vi "Get Data content.vi"(4 "error in (no error)":errorcluster, 6 "Data in":refnum<class "Data.lvclass">) -> (0 "error out":errorcluster, 2 "Data out":refnum<class "Data.lvclass">, 3 "Data Content":sgl[][](array[numeric]))   [LabVIEW 2017]
doc: "Displays the content of a Data object containing 2-dimensional OCT data, in an intensity graph. The refractive index can be specified to account for skew in the z axis.\nThe raw image data is returned in a 2D array of single."
uses:
  C:/Program Files/Thorlabs/SpectralRadar/LabVIEW/2012/user.lib/SpectralRadar.llb/Data.lvclass
  C:/Program Files/Thorlabs/SpectralRadar/LabVIEW/2012/user.lib/SpectralRadar.llb/Data Property Int Selection.ctl
  C:/Program Files/Thorlabs/SpectralRadar/LabVIEW/2012/user.lib/SpectralRadar.llb/get Data Property Int.vi
  SpectralRadar.dll
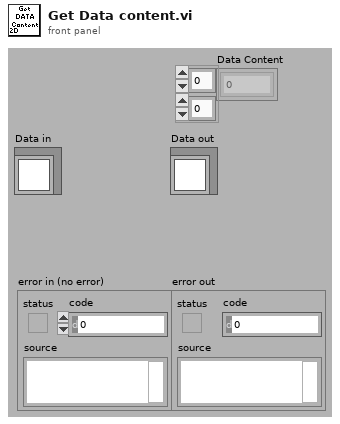
[diagram p1: front panel]
types:
  T1 = typedef "Data.lvclass/Data Property Int Selection.ctl" = enum16{"Dimensions", "Size 1", "Size 2", "Size 3", "Number of Data Points", "Data Size in Bytes", "Bytes per Pixel"}
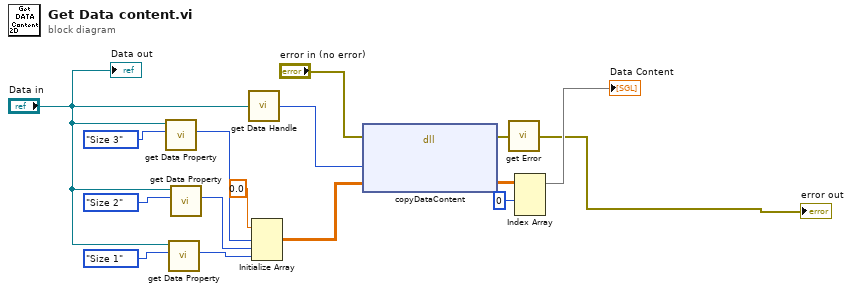
[diagram p0: block diagram]
diagram:
  n1 = call-poly "get Data Property.vi"("Data Property Selection"=Data_Property_Int_Selection."Size 3", "Data"="Data in") -> ("Property Value"=w3:i32)  [unwired: 3 in, 2 out]
  n2 = call-poly "get Data Property.vi"("Data Property Selection"=Data_Property_Int_Selection."Size 1", "Data"="Data in") -> ("Property Value"=w9:i32)  [unwired: 3 in, 2 out]
  n3 = call-poly "get Data Property.vi"("Data Property Selection"=Data_Property_Int_Selection."Size 2", "Data"="Data in") -> ("Property Value"=w8:i32)  [unwired: 3 in, 2 out]
  n4 = call "get Data Handle.vi"("Data"="Data in") -> ("Handle"=w15:u64)
  n5 = Initialize Array(sgl 0.0 ("element"), w3, w8, w9) -> (w14:sgl[][][])
  n6 = dll-call lib="SpectralRadar.dll" fn="copyDataContent"(error in="error in (no error)", "Data Handle"=w15, "Data Content"=w14) -> (error out=w7:errorcluster, "Data Content"=w13:sgl[][][])  [unwired: 4 in, 1 out]
  n7 = call "get Error.vi"("error in (no error)"=w7) -> ("error out"=→"error out":errorcluster)
  n8 = Index Array(array=w13, index (dim 0)=0 ("index (page)")) -> (element=→"Data Content":sgl[][])  [unwired: 2 in]
  "Data out" <- "Data in"
